vi "Plink.vi"(8 "error in":errorcluster, 9 "Command(s) to Execute":string="pwd", 10 "Host":string="172.22.11.2", 11 "plink path":path=path "bin/plink.exe") -> (0 "error out":errorcluster, 1 "return code":i32, 2 "Errors":string, 3 "Command Return Value(s)":string, 5 "Command Executed":string)   [LabVIEW 2016]
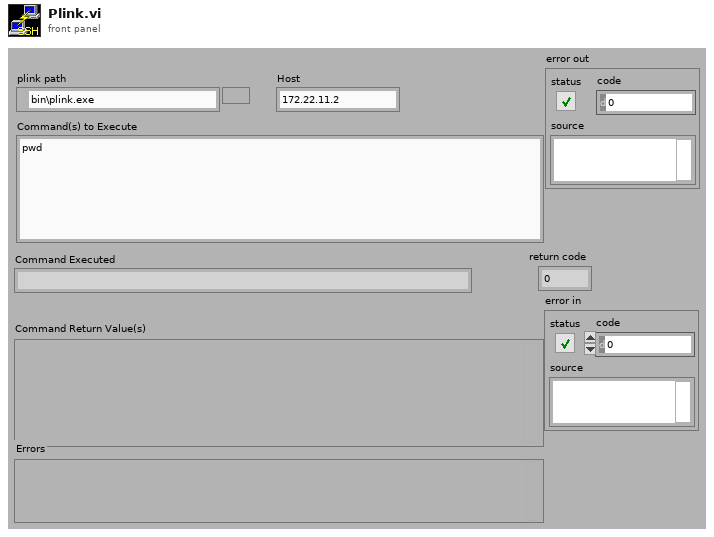
[diagram p1: front panel]
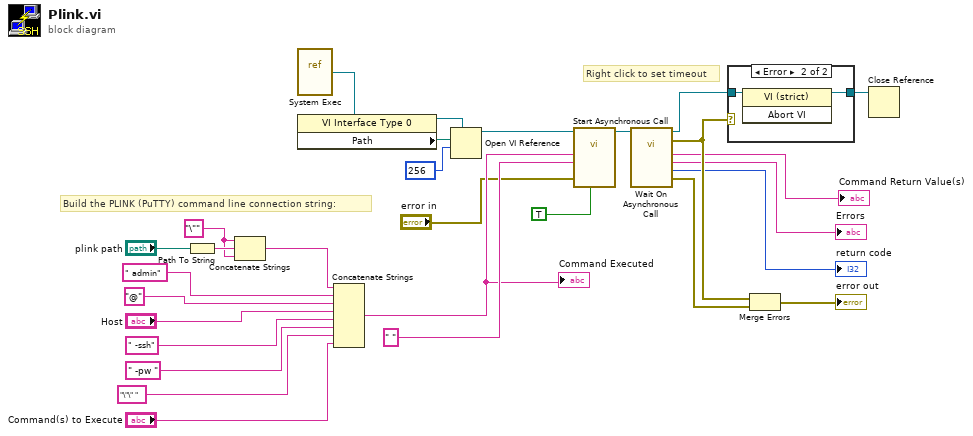
[diagram p0: block diagram]
diagram:
  w20 = "\"" ("string")
  # "Right click to set timeout"
  # "Build the PLINK (PuTTY) command line connection string:"
  n1 = Path To String(path="plink path") -> (string=w21:string)
  n2 = Concatenate Strings(w20, w21, w20) -> (w19:string)
  n3 = vi-ref <vilib>:"System Exec.vi"() -> (w17:refnum<vi>)
  n4 = property class="VI Interface Type 0"(reference=w17) -> (reference out=w14:refnum<vi>, "Path"=w16:path)  [unwired: 1 in, 1 out]
  n5 = Concatenate Strings(w19, " admin" ("Username"), "@" ("string"), "Host", " -ssh", " -pw " ("string"), "\"\" " ("Password"), "Command(s) to Execute") -> (w2:string)
  "Command Executed" <- w2
  n6 = Open VI Reference(type specifier VI Refnum (for type only)=w14, vi path=w16, options=256) -> (vi reference=w18:refnum<vi>)  [unwired: 3 in, 1 out]
  n7 = call-by-ref "Start Asynchronous Call"(reference=w18, "run minimized? (F)"=TRUE ("Hide DOS\nWindow?"), "error in (no error)"="error in", "standard input"=" ", "command line"=w2) -> (reference out=w13:refnum<vi>)  [unwired: 5 in, 5 out]
  n8 = call-by-ref "Wait On Asynchronous Call"(reference=w13) -> (reference out=w8:refnum<vi>, error out=w7:errorcluster, 0:"error out"=w10:errorcluster, "return code"=→"return code":i32, "standard error"=→"Errors":string, "standard output"=→"Command Return Value(s)":string)  [unwired: 9 in]
  n9 = case shown="Error" w7 {
    tunnel: [w30 w32] -> w9
    tunnel: w8 -> [w30 w31]
    frame No Error {
    }
    frame Error {
      n10 = invoke class="VI (strict)" method="Abort VI"(reference=w31) -> (reference out=w32:refnum<vi>)  [unwired: 2 in, 2 out]
    }
  }
  n11 = Merge Errors(w7, w10) -> (→"error out":errorcluster)
  n12 = Close Reference(reference=w9) -> ()  [unwired: 1 in, 1 out]
